vi "Factory settings laden FT-IR Parameter.vi"(8 "error in (no error)":errorcluster caption="Fehler (Eingang, kein Fehler)", 9 "Dateiname":string="abc", 11 "Ordner des Haupt-VIs":path) -> (0 "error out":errorcluster caption="Fehler (Ausgang)")   [LabVIEW 2020, in "allgemeine Sub-VIs.lvlib"]
uses:
  allgemeine Sub-VIs.lvlib
  Seiten/FT-IR/FGV FT-IR Diagnose Aktionen.ctl
  <vilib>/Utility/config.llb/Read Key (U32).vi
  <vilib>/Utility/config.llb/Read Key (String).vi
  <vilib>/Utility/config.llb/Read Key (Boolean).vi
  <vilib>/Utility/config.llb/Read Key (Path).vi
  <vilib>/Utility/config.llb/Read Key (Double).vi
  <vilib>/Utility/config.llb/NI_LVConfig.lvlib
  Seiten/FT-IR/FT-IR.lvlib
panel:
  out "NoOfGases":u32
  out "NoOfScan":u32
  out "CurrentRecipe":string
  out "labEnabled":bool
  out "labPath":path
  out "labBaseName":string
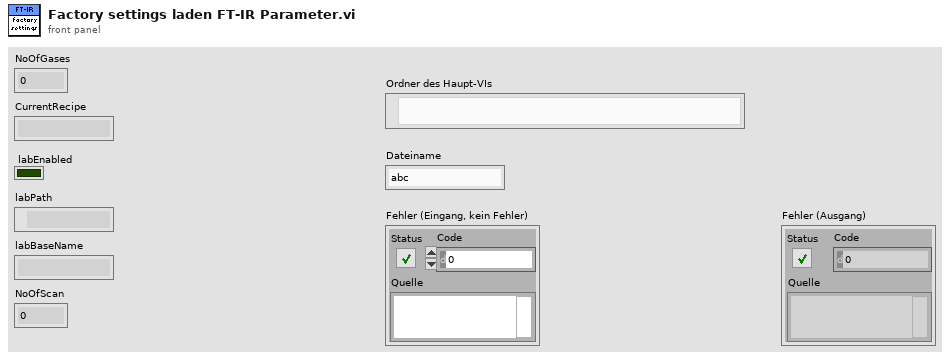
[diagram p1: front panel]
types:
  T1 = typedef "FT-IR.lvlib/FGV FT-IR Diagnose Aktionen.ctl" = enum16{"Lesen", "Diagnose Schreiben", "Min Schreiben", "Max Schreiben"}
  T2 = typedef "NI_LVConfig.lvlib/Config Data RefNum.ctl" = refnum<k1>
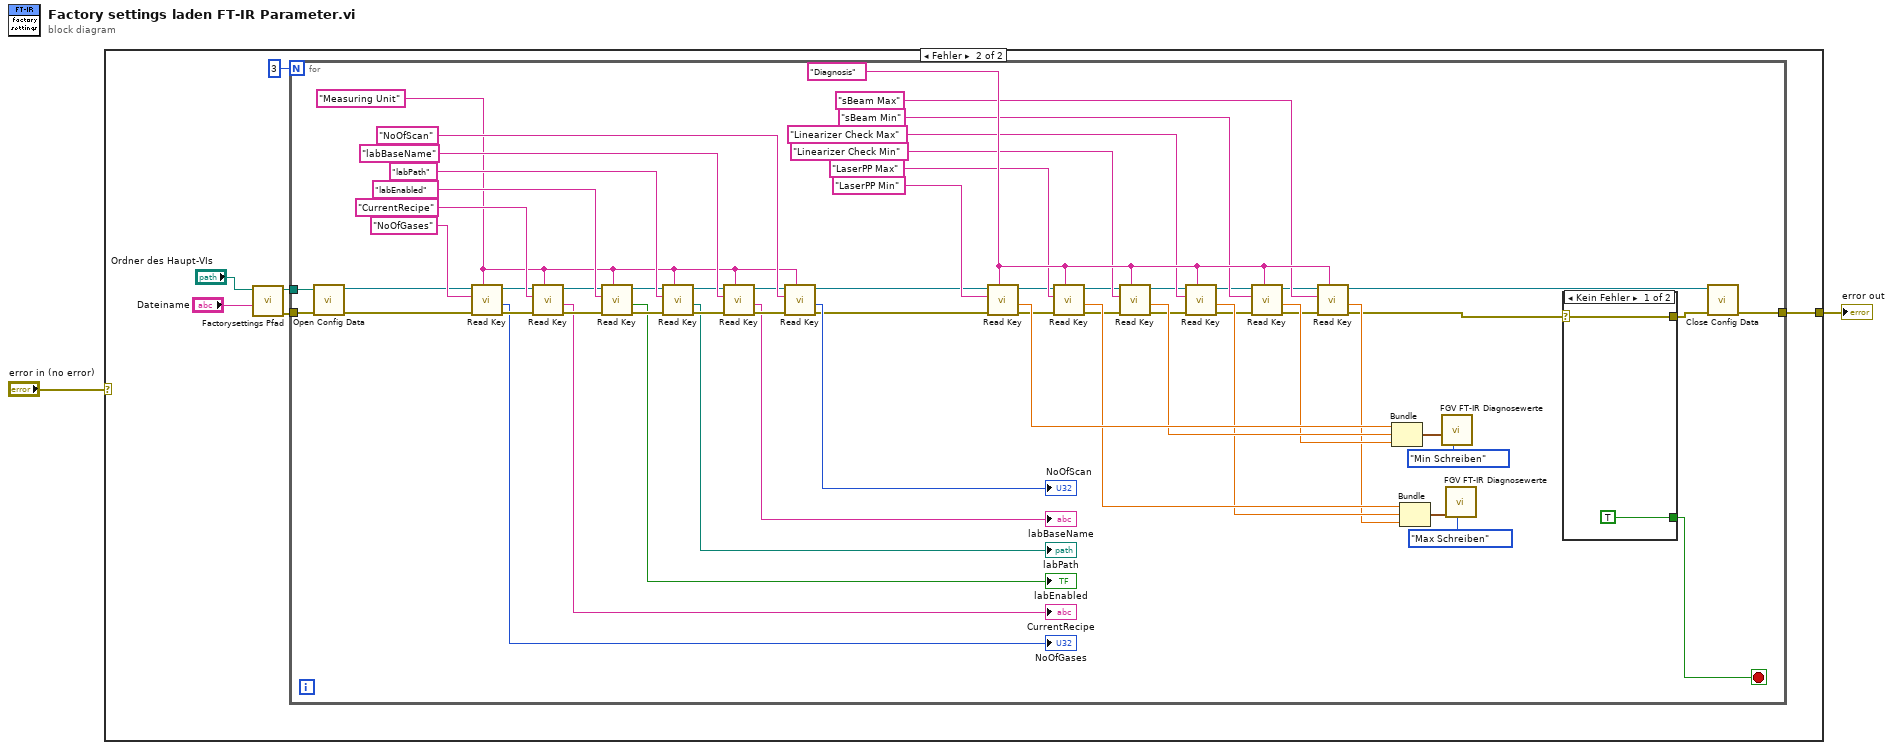
[diagram p0: block diagram]
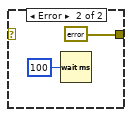
[diagram p3: hidden frame]
diagram:
  n1 = case shown="Fehler" "error in (no error)" {
    selector: "error in (no error)" -> [w3 _]
    tunnel: [w3 w9] -> w1
    frame No Error {
    }
    frame Error {
      n2 = call "Factorysettings Pfad.vi"("Dateiname"="Dateiname", "Ordner des Haupt-VIs"="Ordner des Haupt-VIs") -> ("error out"=w7:errorcluster, "Pfad Factorysettings"=w8:path)  [unwired: 8 in]
      n3 = for {
        N: 3 -> [_]
        tunnel: w8 -> [w52]
        tunnel: w7 -> [w51]
        tunnel: [w53] -> w9
        stop <- w10 stop-if-true
        w60 = "Diagnosis" ("section")
        w61 = "Measuring Unit" ("section")
        n4 = call <vilib>:"Open Config Data.vi"("error in (no error)"=w51, "configuration file path"=w52) -> ("error out"=w66:errorcluster, "refnum"=w67:T2)  [unwired: 7 in, 1 out]
        n5 = call-poly <vilib>:"Read Key.vi"("section"=w61, "error in (no error)"=w66, "key"="NoOfGases", "refnum"=w67) -> ("error out"=w50:errorcluster, "value"=→"NoOfGases":u32, "refnum out"=w49:T2)  [unwired: 4 in, 1 out]
        n6 = call-poly <vilib>:"Read Key.vi"("section"=w61, "error in (no error)"=w50, "key"="CurrentRecipe", "refnum"=w49) -> ("error out"=w48:errorcluster, "value"=→"CurrentRecipe":string, "refnum out"=w47:T2)  [unwired: 4 in, 1 out]
        n7 = call-poly <vilib>:"Read Key.vi"("section"=w61, "error in (no error)"=w48, "key"="labEnabled", "refnum"=w47) -> ("error out"=w46:errorcluster, "value"=→"labEnabled":bool, "refnum out"=w45:T2)  [unwired: 4 in, 1 out]
        n8 = call-poly <vilib>:"Read Key.vi"("section"=w61, "error in (no error)"=w46, "key"="labPath", "refnum"=w45) -> ("error out"=w44:errorcluster, "value"=→"labPath":path, "refnum out"=w43:T2)  [unwired: 4 in, 1 out]
        n9 = call-poly <vilib>:"Read Key.vi"("section"=w61, "error in (no error)"=w44, "key"="labBaseName", "refnum"=w43) -> ("error out"=w41:errorcluster, "value"=→"labBaseName":string, "refnum out"=w42:T2)  [unwired: 4 in, 1 out]
        n10 = call-poly <vilib>:"Read Key.vi"("section"=w61, "error in (no error)"=w41, "key"="NoOfScan", "refnum"=w42) -> ("error out"=w13:errorcluster, "value"=→"NoOfScan":u32, "refnum out"=w14:T2)  [unwired: 4 in, 1 out]
        n11 = call-poly <vilib>:"Read Key.vi"("section"=w60, "error in (no error)"=w13, "key"="LaserPP Min", "refnum"=w14) -> ("error out"=w19:errorcluster, "value"=w32:dbl, "refnum out"=w24:T2)  [unwired: 4 in, 1 out]
        n12 = call-poly <vilib>:"Read Key.vi"("section"=w60, "error in (no error)"=w19, "key"="LaserPP Max", "refnum"=w24) -> ("error out"=w18:errorcluster, "value"=w28:dbl, "refnum out"=w23:T2)  [unwired: 4 in, 1 out]
        n13 = call-poly <vilib>:"Read Key.vi"("section"=w60, "error in (no error)"=w18, "key"="Linearizer Check Min", "refnum"=w23) -> ("error out"=w17:errorcluster, "value"=w30:dbl, "refnum out"=w22:T2)  [unwired: 4 in, 1 out]
        n14 = call-poly <vilib>:"Read Key.vi"("section"=w60, "error in (no error)"=w17, "key"="Linearizer Check Max", "refnum"=w22) -> ("error out"=w16:errorcluster, "value"=w27:dbl, "refnum out"=w21:T2)  [unwired: 4 in, 1 out]
        n15 = call-poly <vilib>:"Read Key.vi"("section"=w60, "error in (no error)"=w16, "key"="sBeam Min", "refnum"=w21) -> ("error out"=w15:errorcluster, "value"=w29:dbl, "refnum out"=w20:T2)  [unwired: 4 in, 1 out]
        n16 = call-poly <vilib>:"Read Key.vi"("section"=w60, "error in (no error)"=w15, "key"="sBeam Max", "refnum"=w20) -> ("error out"=w12:errorcluster, "value"=w26:dbl, "refnum out"=w70:T2)  [unwired: 4 in, 1 out]
        n17 = Bundle("value"=w32, "value"=w30, "value"=w29) -> (w31:cluster{"value":dbl, "value":dbl, "value":dbl})  [unwired: 1 in]
        n18 = Bundle("value"=w28, "value"=w27, "value"=w26) -> (w25:cluster{"value":dbl, "value":dbl, "value":dbl})  [unwired: 1 in]
        n19 = call "FGV FT-IR Diagnosewerte.vi"("Aktionen"=FGV_FT-IR_Diagnose_Aktionen."Min Schreiben", "FT-IR MIN"=w31) -> ()  [unwired: 4 in, 6 out]
        n20 = call "FGV FT-IR Diagnosewerte.vi"("Aktionen"=FGV_FT-IR_Diagnose_Aktionen."Max Schreiben", "FT-IR MAX"=w25) -> ()  [unwired: 4 in, 6 out]
        n21 = case shown="Kein Fehler" w12 {
          selector: w12 -> [w72 _]
          tunnel: [w72 errorcluster {"status"=FALSE, "code"=0, "source"=""} ("error IO")] -> w11
          tunnel: [TRUE _] -> w10
          frame No Error {
          }
          frame Error {
            n22 = Wait (ms)(milliseconds to wait=u32 100 ("Zu wartende ms")) -> ()  [unwired: 1 out]
          }
        }
        n23 = call <vilib>:"Close Config Data.vi"("error in (no error)"=w11, "refnum"=w70) -> ("error out"=w53:errorcluster)  [unwired: 8 in, 1 out]
      }
    }
  }
  "error out" <- w1
